vi "Read alarm XML.vi"(11 "模块名称":string) -> (3 "报警输出":string[][](array[string]))   [LabVIEW 2016, in "质控单元V1.lvlib"]
uses:
  <vilib>/Utility/xml.llb/Write to XML File(string).vi
  <vilib>/Utility/xml.llb/Read From XML File(string).vi
panel:
  in  "报警常量":string[][](array[string])=[["1", "1066", "液位异常告警", "1、建议排查通信是否正常\n2、供电情况是否正常"], ["2", "1067", "柱塞泵故障告警", "1、建议排查通信是否正常\n2、供电情况是否正常"], ["3", "1068", "流程中断告警", ""]]
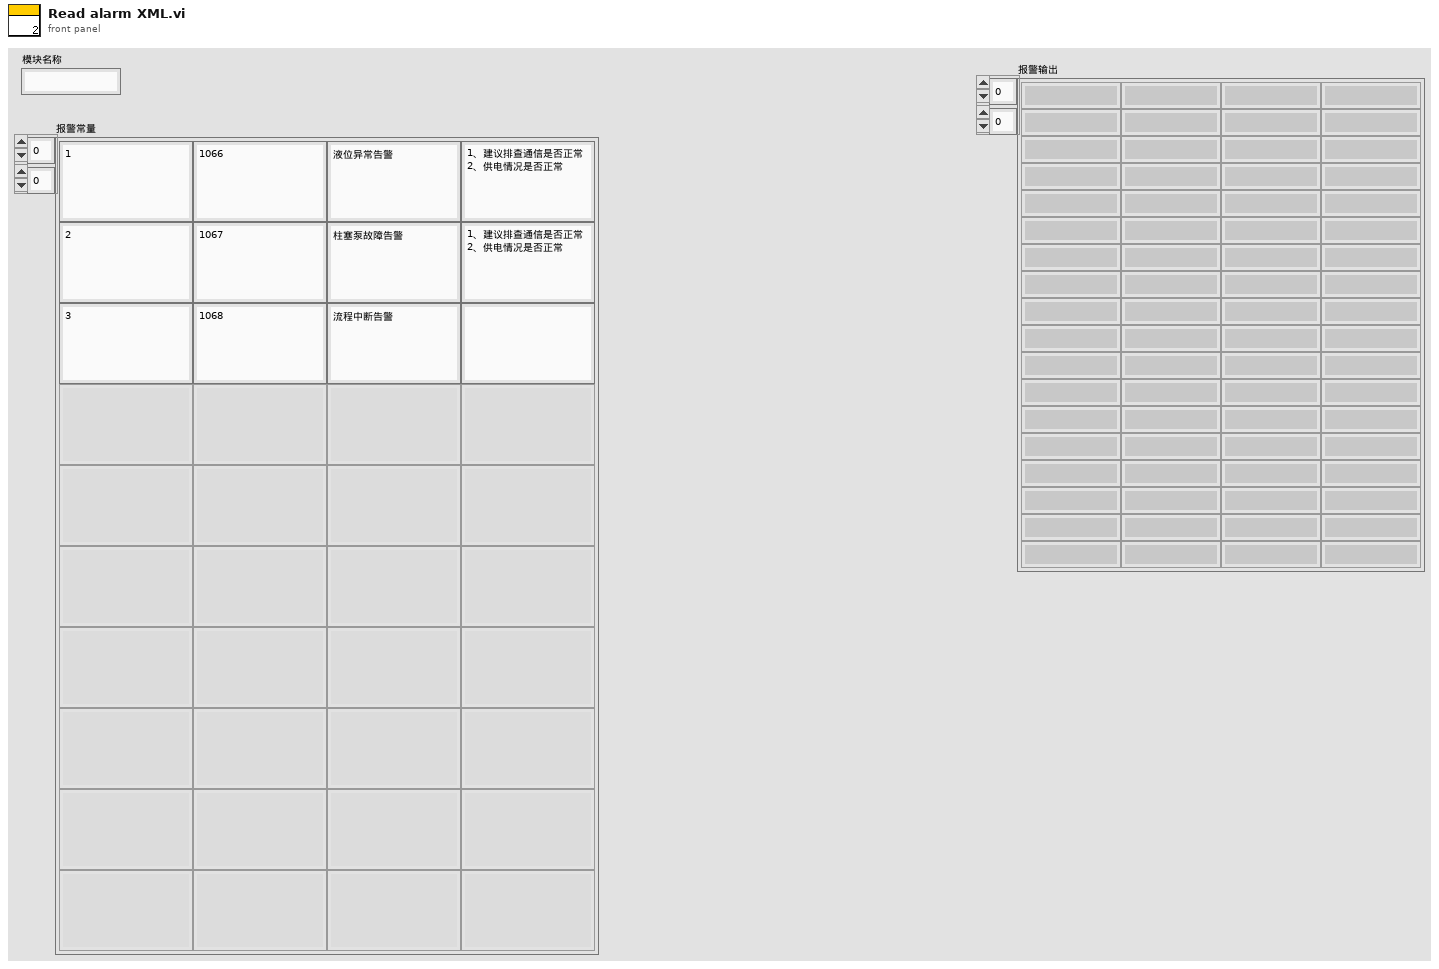
[diagram p1: front panel]
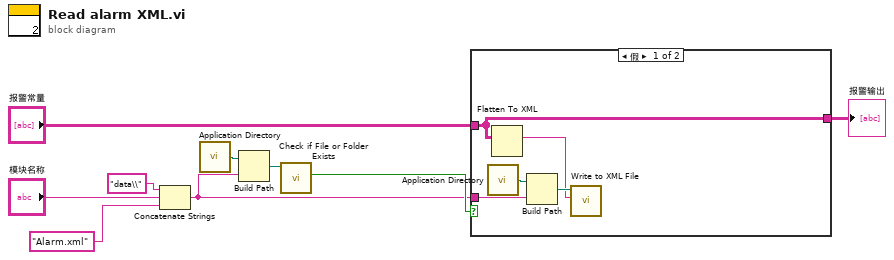
[diagram p0: block diagram]
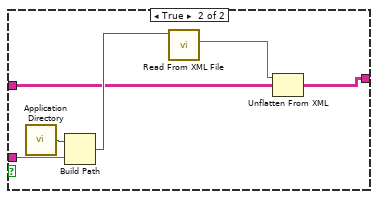
[diagram p2: hidden frame]
diagram:
  n1 = Concatenate Strings("data\\" ("字符串"), "模块名称", "Alarm.xml" ("名称或相对路径")) -> (w6:string)
  n2 = call <vilib>:"Application Directory.vi"() -> ("Application Directory"=w4:path)
  n3 = Build Path(base path=w4, name or relative path=w6) -> (appended path=w5:path)
  n4 = call <vilib>:"Check if File or Folder Exists.vi"("path"=w5) -> ("file or folder exists?"=w7:bool)  [unwired: 8 in, 2 out]
  n5 = case shown="假" w7 {
    tunnel: [w10 w17] -> w8
    tunnel: w6 -> [w11 w16]
    tunnel: "报警常量" -> [w10 w15]
    frame False {
      n6 = call <vilib>:"Application Directory.vi"() -> ("Application Directory"=w13:path)
      n7 = Flatten To XML(anything=w10) -> (xml string=w12:string)
      n8 = Build Path(base path=w13, name or relative path=w11) -> (appended path=w14:path)
      n9 = call-poly <vilib>:"Write to XML File.vi"("XML Input"=w12, "XML File Path"=w14) -> ()  [unwired: 7 in, 3 out]
    }
    frame True {
      n10 = call <vilib>:"Application Directory.vi"() -> ("Application Directory"=w19:path)
      n11 = Build Path(base path=w19, name or relative path=w16) -> (appended path=w18:path)
      n12 = call-poly <vilib>:"Read From XML File.vi"("XML File Path"=w18) -> ("XML Elements"=w20:string)  [unwired: 8 in, 2 out]
      n13 = Unflatten From XML(xml string=w20, type=w15) -> (value=w17:string[][])  [unwired: 1 in, 1 out]
    }
  }
  "报警输出" <- w8
